vi "Create Summary Page.vi"(7 "Summary Data":string[][](array[string]), 8 "error in (no error)":errorcluster, 11 "Report In":refnum<class "NI_report.lvclass">) -> (0 "error out":errorcluster, 3 "Report Out":refnum<class "NI_report.lvclass">)   [LabVIEW 2014]
uses:
  <vilib>/Utility/NIReport.llb/NI_report.lvclass
  <vilib>/addons/_office/excel.llb/Excel Easy Table (str).vi
  <vilib>/addons/_office/NI_ReportGenerationToolkit.lvlib
  <vilib>/Utility/NIReport.llb/Excel/NI_Excel.lvclass
panel:
  in  "Start Cell":cluster{"row":i32, "column":i32}={"row"=3, "column"=0}
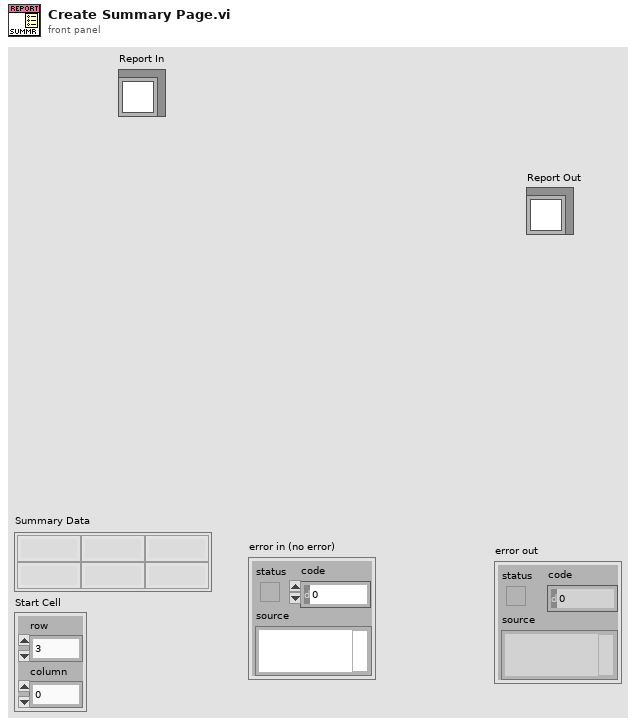
[diagram p1: front panel]
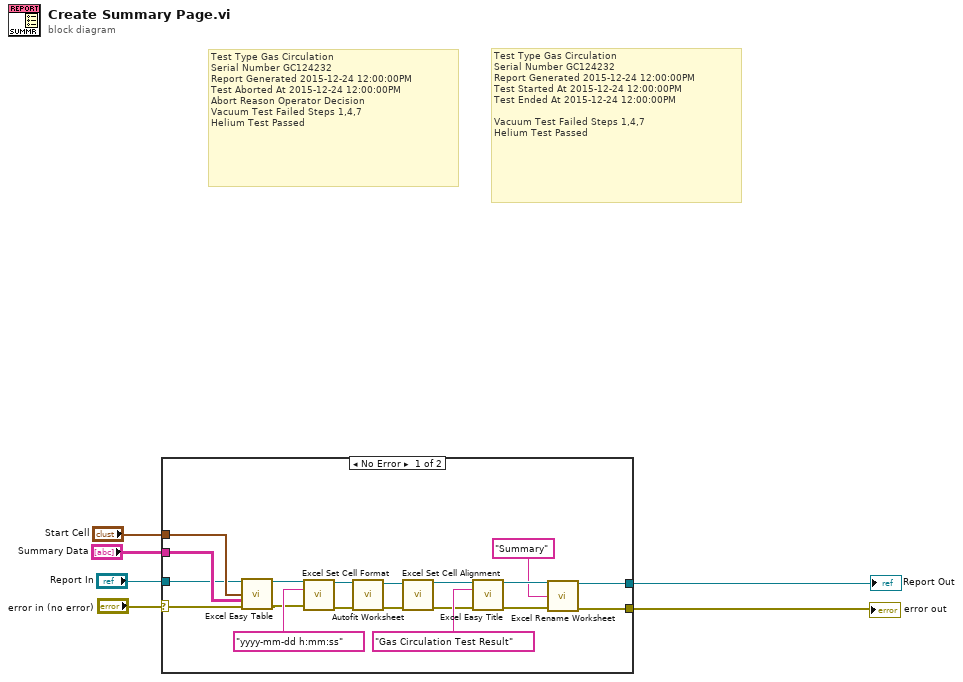
[diagram p0: block diagram]
diagram:
  # "Test Type\tGas Circulation \nSerial Number\tGC124232\nReport Generated\t2015-12-24 12:00:00PM\nTest Started At\t2015-12-24 12:00:00PM\nTest Ended At\t2015-12-24 12:00:00PM\n\nVacuum Test\tFailed Steps 1,4,7\nHelium Test\tPassed"
  # "Test Type\tGas Circulation \nSerial Number\tGC124232\nReport Generated\t2015-12-24 12:00:00PM\nTest Aborted At\t2015-12-24 12:00:00PM\nAbort Reason\tOperator Decision\nVacuum Test\tFailed Steps 1,4,7\nHelium Test\tPassed"
  n1 = case shown="No Error" "error in (no error)" {
    selector: "error in (no error)" -> [w22 w27]
    tunnel: [w7 w27] -> w6
    tunnel: "Report In" -> [w23 w26]
    tunnel: [w8 w26] -> w3
    tunnel: "Start Cell" -> [w25 _]
    tunnel: "Summary Data" -> [w24 _]
    frame No Error {
      n2 = call-poly <vilib>:"Excel Easy Table.vi"("report in"=w23, "start (0, 0)"=w25, "text data"=w24, "error in (no error)"=w22) -> ("report out"=w20:refnum<class "NI_report.lvclass">, "error out"=w19:errorcluster)  [unwired: 7 in, 3 out]
      n3 = call <vilib>:"Excel Set Cell Format.vi"("report in"=w20, "number format"="yyyy-mm-dd h:mm:ss", "error in (no error)"=w19) -> ("report out"=w17:refnum<class "NI_report.lvclass">, "error out"=w18:errorcluster)  [unwired: 11 in]
      n4 = call "Autofit Worksheet.vi"("error in (no error)"=w18, "Report In"=w17) -> ("error out"=w15:errorcluster, "Report Out"=w14:refnum<class "NI_report.lvclass">)  [unwired: 8 in]
      n5 = call <vilib>:"Excel Set Cell Alignment.vi"("report in"=w14, "error in (no error)"=w15) -> ("report out"=w13:refnum<class "NI_report.lvclass">, "error out"=w12:errorcluster)  [unwired: 12 in]
      n6 = call <vilib>:"Excel Easy Title.vi"("report in"=w13, "title"="Gas Circulation Test Result", "error in (no error)"=w12) -> ("report out"=w11:refnum<class "NI_report.lvclass">, "error out"=w10:errorcluster)  [unwired: 10 in, 1 out]
      n7 = call <vilib>:"Excel Rename Worksheet.vi"("report in"=w11, "worksheet name (\"\")"="Summary" ("worksheet name (\"\")"), "error in (no error)"=w10) -> ("report out"=w8:refnum<class "NI_report.lvclass">, "error out"=w7:errorcluster)  [unwired: 11 in]
    }
    frame Error {
    }
  }
  "error out" <- w6
  "Report Out" <- w3
